vi "IntakeUntilBall.vi"() -> ()   [LabVIEW 2018]
panel:
  in  "AbortTime":dbl=4.0
  in  "NoWait":bool
  in  "Speed":dbl=1.0
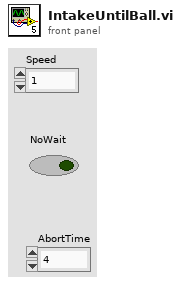
[diagram p1: front panel]
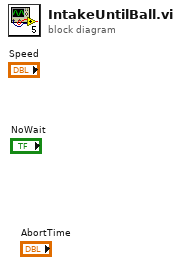
[diagram p0: block diagram]
diagram:
